vi "DFConfig My.Datafinder.vi"(8 "error in (no error)":errorcluster, 10 "Spartan Data Path (\"\")":path, 11 "My.DataFinder In":string) -> (0 "error out":errorcluster, 3 "My.DataFinder Out":string)   [LabVIEW 2011]
uses:
  DFConfig GLOBAL.ctl
  DFConfig SEARCH AREA.ctl
  DFConfig INDEXER.ctl
  <vilib>/Utility/miscctls.llb/LVDateTimeRec.ctl
  ITK EXT/utils/strutil.llb/Case Matching.ctl
  server lib/Spartan CONFIG Global.vi
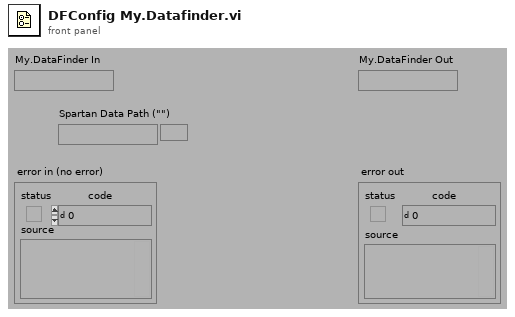
[diagram p1: front panel]
types:
  T1 = typedef "Case Matching.ctl" = enum16{"a != A", "a == A", "system"}
  T2 = typedef "LVDateTimeRec.ctl" = cluster{"fractional second":dbl, "second":i32, "minute":i32, "hour":i32, "day of month":i32, "month":i32, "year":i32, "day of week":i32, "day of year":i32, "DST":i32}
  T3 = typedef "DFConfig INDEXER.ctl" = cluster{"repeat":enum16{"hourly", "daily", "weekly", "never"}, "enable_observer":bool, "starttime":timestamp, "timeout":i32}
  T4 = typedef "DFConfig SEARCH AREA.ctl" = cluster{"path":path, "remotepath":path, "alias":string, "volatile":bool, "type":string, "lastcrawl":timestamp, "numberofcrawls":i32, "crawlnow":bool}
  T5 = typedef "DFConfig GLOBAL.ctl" = cluster{"Query Timeout (120)":i32, "Connection Timeout (30)":i32, "Indexer Idle Time (10)":i32, " Database Path (empty)":path}
  T6 = typedef "Keyed Array.ctl" = cluster{"keys":string[], "values":string[]}
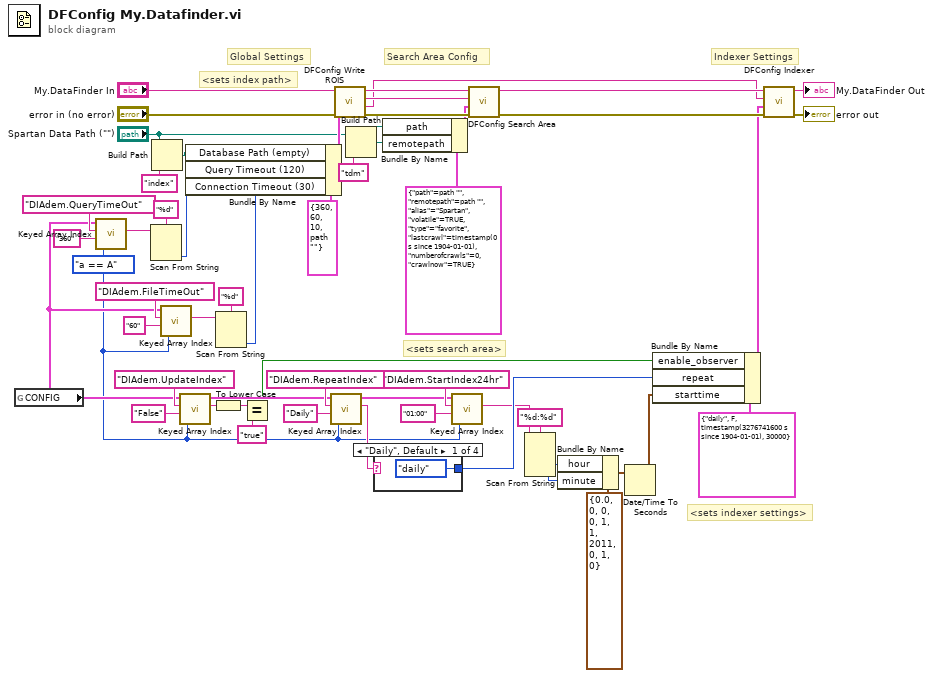
[diagram p0: block diagram]
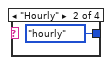
[diagram p2: hidden frame]
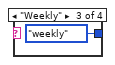
[diagram p3: hidden frame]
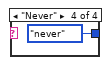
[diagram p4: hidden frame]
diagram:
  w1 = Case_Matching."a == A" ("case matching (sensitive)")
  # "<sets indexer settings>"
  # "<sets search area>"
  # "<sets index path>"
  # "Indexer Settings"
  # "Search Area Config"
  # "Global Settings"
  n1 = global read "Spartan CONFIG Global.vi" "CONFIG"() -> (w4:T6)
  n2 = call "Keyed Array Index.vi"("case matching (sensitive)"=w1, "default value"="360", "key"="DIAdem.QueryTimeOut", "array in"=w4) -> ("value"=w9:string)  [unwired: 3 out]
  n3 = Scan From String(format string="%d" ("regular expression"), input string=w9) -> (output 1=w8:i32)  [unwired: 3 in, 3 out]
  n4 = Build Path(base path="Spartan Data Path (\"\")", name or relative path="index") -> (appended path=w41:path)
  n5 = call "Keyed Array Index.vi"("case matching (sensitive)"=w1, "default value"="60", "key"="DIAdem.FileTimeOut", "array in"=w4) -> ("value"=w7:string)  [unwired: 3 out]
  n6 = call "Keyed Array Index.vi"("case matching (sensitive)"=w1, "default value"="False", "key"="DIAdem.UpdateIndex", "array in"=w4) -> ("value"=w31:string, "duplicate array"=w26:T6)  [unwired: 2 out]
  n7 = To Lower Case(string=w31) -> (all lower case string=w30:string)
  n8 = Scan From String(format string="%d" ("regular expression"), input string=w7) -> (output 1=w2:i32)  [unwired: 3 in, 3 out]
  n9 = Bundle By Name(cluster=T5 {"Query Timeout (120)"=360, "Connection Timeout (30)"=60, "Indexer Idle Time (10)"=10, " Database Path (empty)"=path ""} ("Global Settings"), "Database Path (empty)"=w41, "Query Timeout (120)"=w8, "Connection Timeout (30)"=w2) -> (w37:T5)
  n10 = Equal?(x=w30, y="true" ("default value")) -> (x = y?=w24:bool)
  n11 = call "Keyed Array Index.vi"("case matching (sensitive)"=w1, "default value"="Daily", "key"="DIAdem.RepeatIndex", "array in"=w26) -> ("value"=w25:string, "duplicate array"=w21:T6)  [unwired: 2 out]
  n12 = call "DFConfig Write ROIS.vi"("error in (no error)"="error in (no error)", "Global Settings"=w37, "My.DataFinder In"="My.DataFinder In") -> ("error out"=w52:errorcluster, "CrawlSettings ID"=w48:string, "First CrawlDir ID"=w53:string, "My.DataFinder Out"=w54:string)  [unwired: 5 out]
  n13 = Build Path(base path="Spartan Data Path (\"\")", name or relative path="tdm") -> (appended path=w39:path)
  n14 = case shown="\"Daily\", Default" w25 {
    tunnel: [enum16{"hourly", "daily", "weekly", "never"}."daily" ("repeat") enum16{"hourly", "daily", "weekly", "never"}."hourly" ("repeat") enum16{"hourly", "daily", "weekly", "never"}."weekly" ("repeat") enum16{"hourly", "daily", "weekly", "never"}."never" ("repeat")] -> w20
    frame "Daily", Default {
    }
    frame "Hourly" {
    }
    frame "Weekly" {
    }
    frame "Never" {
    }
  }
  n15 = Bundle By Name(cluster=T4 {"path"=path "", "remotepath"=path "", "alias"="Spartan", "volatile"=TRUE, "type"="favorite", "lastcrawl"=timestamp(0 s since 1904-01-01), "numberofcrawls"=0, "crawlnow"=TRUE} ("Datafinder Search Area"), "path"=w39, "remotepath"=w39) -> (w38:T4)
  n16 = call "Keyed Array Index.vi"("case matching (sensitive)"=w1, "default value"="01:00", "key"="DIAdem.StartIndex24hr", "array in"=w21) -> ("value"=w19:string)  [unwired: 3 out]
  n17 = call "DFConfig Search Area.vi"("error in (no error)"=w52, "Datafinder Search Area"=w38, "CrawlDir ID (\"\")"=w53, "My.DataFinder In"=w54) -> ("error out"=w51:errorcluster, "My.DataFinder Out"=w50:string)  [unwired: 6 out]
  n18 = Scan From String(format string="%d:%d" ("regular expression"), input string=w19) -> (output 1=w16:i32, output 2=w15:i32)  [unwired: 4 in, 3 out]
  n19 = Bundle By Name(cluster=T2 {"fractional second"=0.0, "second"=0, "minute"=0, "hour"=0, "day of month"=1, "month"=1, "year"=2011, "day of week"=0, "day of year"=1, "DST"=0} ("date time rec"), "hour"=w16, "minute"=w15) -> (w14:T2)
  n20 = Date/Time To Seconds(2:w14) -> (0:w13:timestamp)  [unwired: 1 in]
  n21 = Bundle By Name(cluster=T3 {"repeat"=enum."daily", "enable_observer"=FALSE, "starttime"=timestamp(3276741600 s since 1904-01-01), "timeout"=30000} ("Datafinder Indexer"), "enable_observer"=w24, "repeat"=w20, "starttime"=w13) -> (w32:T3)
  n22 = call "DFConfig Indexer.vi"("error in (no error)"=w51, "Datafinder Indexer"=w32, "CrawlSettings ID (\"\")"=w48, "My.DataFinder In"=w50) -> ("error out"=→"error out":errorcluster, "My.DataFinder Out"=→"My.DataFinder Out":string)  [unwired: 6 out]
